vi "RT Driver_Set Date And Time.vi"(4 "Password":string, 6 "User name":string, 8 "error in (no error)":errorcluster, 9 "Configuration":T1={"Server IP Address"="206.246.122.250", "UDP Port"=123, "Synchronization Interval"=60.0, "Synchronization Threshold"=0.01, "Debug Output Strings"=TRUE, "Maximum Offset To Apply"=0.0}, 10 "New time zone (Leave blank to keep current time zone)":string, 11 "Correction (S/s)":dbl) -> (0 "error out":errorcluster)   [LabVIEW 2013, in "SNTP Light Custom Device Engine.lvlib"]
uses:
  SNTP Light Custom Device Engine.lvlib
  RT_Configuration_Data.ctl
  RT Driver_Global.vi
  <vilib>/nisyscfg/nisyscfg.lvlib
  <vilib>/NI_Real-Time Target Support.lvlib
  <vilib>/NI Veristand/Custom Device Tools/Custom Device Utility Library/Custom Device Utility Library.lvlib
panel:
  out "New Time":timestamp format="%<%.6X\n%x>T"
  out "current time":timestamp format="%<%.6X\n%x>T"
  out "Last Correction (s)":dbl
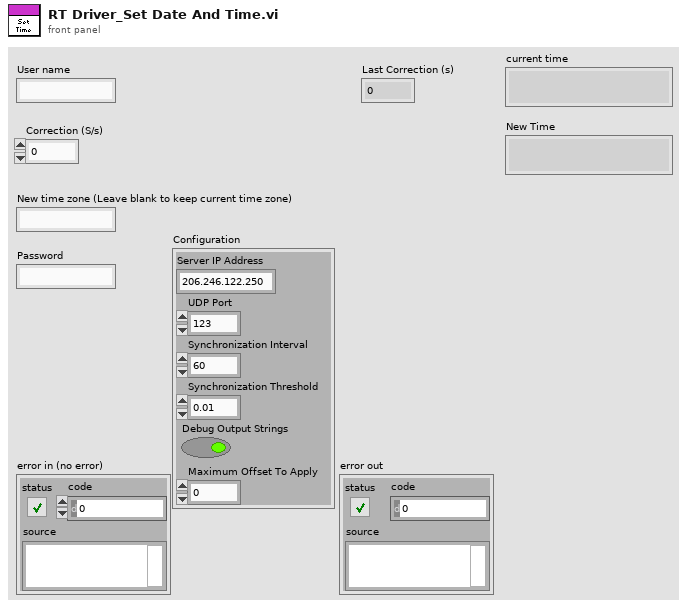
[diagram p1: front panel]
types:
  T1 = typedef "SNTP Light Custom Device Engine.lvlib/RT_Configuration_Data.ctl" = cluster{"Server IP Address":string, "UDP Port":u16, "Synchronization Interval":dbl, "Synchronization Threshold":dbl, "Debug Output Strings":bool, "Maximum Offset To Apply":dbl}
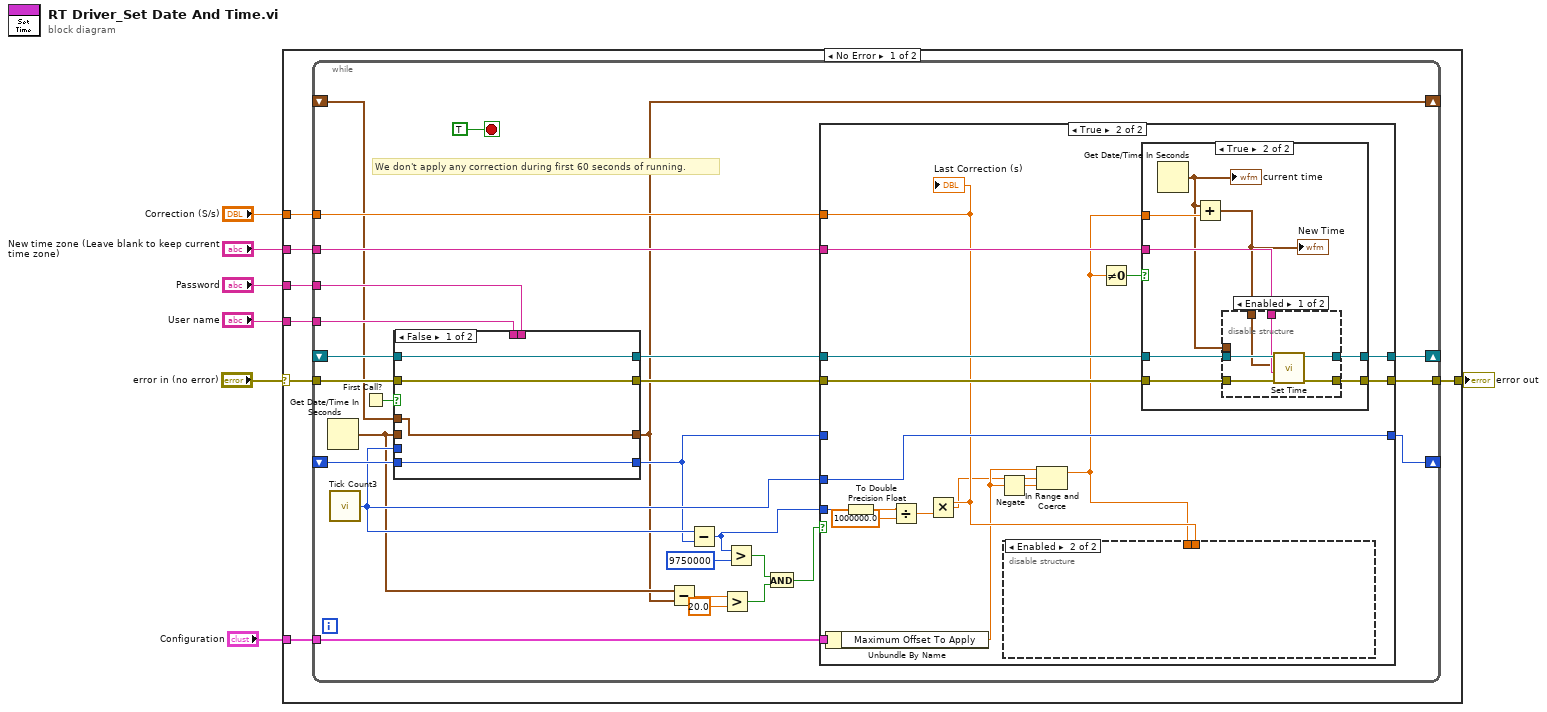
[diagram p0: block diagram]
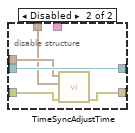
[diagram p4: hidden frame]
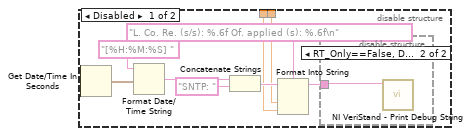
[diagram p5: hidden frame]
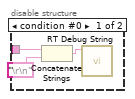
[diagram p6: hidden frame]
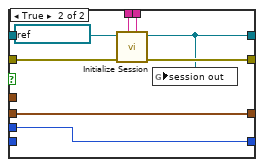
[diagram p7: hidden frame]
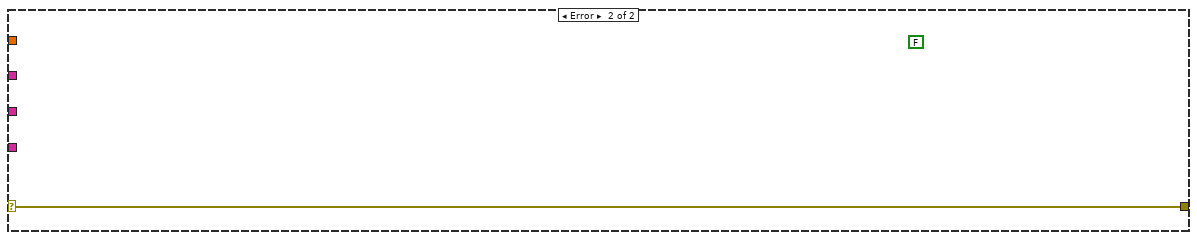
[diagram p8: hidden frame]
diagram:
  n1 = case shown="No Error" "error in (no error)" {
    selector: "error in (no error)" -> [w10 w108]
    tunnel: [w14 w108] -> w7
    tunnel: "Password" -> [w13 _]
    tunnel: "User name" -> [w12 _]
    tunnel: "New time zone (Leave blank to keep current time zone)" -> [w11 _]
    tunnel: "Correction (S/s)" -> [w9 _]
    tunnel: "Configuration" -> [w8 _]
    frame No Error {
      n2 = while {
        tunnel: w11 -> [w39]
        tunnel: w12 -> [w38]
        tunnel: w13 -> [w37]
        tunnel: w10 -> [w36]
        tunnel: [w34] -> w14
        shift-right: [w33] -> _
        shift-left: _ -> [w32]
        tunnel: w9 -> [w30]
        shift-right: [w26] -> _
        shift-left: _ -> [w29]
        shift-right: [w21] -> _
        shift-left: _ -> [w23]
        tunnel: w8 -> [w15]
        stop <- TRUE stop-if-true
        # "We don't apply any correction during first 60 seconds of running."
        n3 = Get Date/Time In Seconds() -> (seconds since 1Jan1904=w22:timestamp)
        n4 = call "Tick Count3"() -> ("Tick Count(uSec)"=w28:u32)
        n5 = First Call?() -> (First Call?: T/F=w31:bool)
        n6 = case shown="False" w31 {
          tunnel: [w99 w102] -> w41
          tunnel: [w98 w107] -> w40
          tunnel: w38 -> [_ w106]
          tunnel: w37 -> [_ w105]
          tunnel: w36 -> [w98 w103]
          tunnel: w32 -> [w99 _]
          tunnel: w29 -> [w97 _]
          tunnel: [w97 w101] -> w27
          tunnel: w28 -> [_ w101]
          tunnel: [w96 w100] -> w21
          tunnel: w22 -> [_ w100]
          tunnel: w23 -> [w96 _]
          frame False {
          }
          frame True {
            n7 = call <vilib>:"Initialize Session.vi"("password"=w105, "user name"=w106, "error in (no error)"=w103, "target (localhost)"=refnum<k21> "localhost" ("Target")) -> ("error out"=w107:errorcluster, "session out"=w102:refnum<k21>)  [unwired: 6 in]
            n8 = global write "RT Driver_Global.vi" "session out"(w102) -> ()
          }
        }
        n9 = Subtract(x=w22, y=w21) -> (x-y=w17:dbl)
        n10 = Subtract(x=w28, y=w27) -> (x-y=w24:u32)
        n11 = Greater?(x=w17, y=20.0) -> (0:w18:bool)
        n12 = Greater?(x=w24, y=u32 9750000) -> (0:w20:bool)
        n13 = And(x=w20, y=w18) -> (x .and. y?=w19:bool)
        n14 = case shown="True" w19 {
          tunnel: w41 -> [w43 w61]
          tunnel: w40 -> [w42 w60]
          tunnel: w39 -> [_ w59]
          tunnel: [w42 w58] -> w34
          tunnel: [w43 w57] -> w33
          tunnel: w28 -> [_ w56]
          tunnel: w27 -> [w44 _]
          tunnel: [w44 w56] -> w26
          tunnel: w24 -> [_ w55]
          tunnel: w30 -> [_ w52]
          tunnel: w15 -> [_ w50]
          frame False {
          }
          frame True {
            n15 = Unbundle By Name(w50) -> ("Maximum Offset To Apply"=w48:dbl)
            n16 = To Double Precision Float(number=w55) -> (double precision float=w53:dbl)
            n17 = Divide(x=w53, y=1000000.0) -> (x/y=w51:dbl)
            n18 = Multiply(x=w52, y=w51) -> (x*y=w46:dbl)
            n19 = Negate(x=w48) -> (-x=w49:dbl)
            n20 = In Range and Coerce(upper limit=w48, x=w46, lower limit=w49) -> (coerced(x)=w45:dbl)  [unwired: 1 out]
            n21 = disable-structure shown="Enabled" {
              disable-tunnel: w52 -> [w85 _]
              disable-tunnel: w45 -> [w84 _]
              frame Disabled {
                n22 = Get Date/Time In Seconds() -> (seconds since 1Jan1904=w87:timestamp)
                n23 = Format Date/Time String(time format string (%c)="[%H:%M:%S] ", seconds (now)=w87) -> (date/time string=w90:string)  [unwired: 1 in]
                n24 = Concatenate Strings(w90, "SNTP: " ("initial string")) -> (w91:string)
                n25 = Format Into String(format string="L. Co. Re. (s/s): %.6f Of. applied (s): %.6f\n", initial string=w91, w85, w84) -> (resulting string=w86:string)  [unwired: 1 in, 1 out]
                n26 = disable-structure shown="RT_Only==False, Default" {
                  disable-tunnel: w86 -> [w94 w95]
                  frame condition #0 {
                    n27 = Concatenate Strings(w94, "\r\n") -> (w93:string)
                    n28 = call <vilib>:"RT Debug String.vi"("String to write"=w93) -> ()  [unwired: 10 in, 1 out]
                  }
                  frame condition #1 (active) {
                    n29 = call <vilib>:"NI VeriStand - Print Debug String.vi"("Message"=w95) -> ()  [unwired: 10 in, 1 out]
                  }
                }
              }
              frame Enabled {
              }
            }
            n30 = Not Equal To 0?(x=w45) -> (x != 0?=w47:bool)
            n31 = case shown="True" w47 {
              tunnel: w61 -> [w63 w71]
              tunnel: w60 -> [w62 w70]
              tunnel: w59 -> [_ w69]
              tunnel: [w62 w67] -> w58
              tunnel: [w63 w66] -> w57
              tunnel: w45 -> [_ w65]
              frame False {
              }
              frame True {
                n32 = Get Date/Time In Seconds() -> (seconds since 1Jan1904=w64:timestamp)
                "current time" <- w64
                n33 = Add(x=w64, y=w65) -> (x+y=w68:timestamp)
                "New Time" <- w68
                n34 = disable-structure shown="Enabled" {
                  disable-tunnel: w71 -> [w77 w82]
                  disable-tunnel: w70 -> [w76 w81]
                  disable-tunnel: w69 -> [w75 _]
                  disable-tunnel: w68 -> [w74 w78]
                  disable-tunnel: [w73 w80] -> w67
                  disable-tunnel: [w72 w82] -> w66
                  disable-tunnel: w64 -> [_ w79]
                  frame Enabled {
                    n35 = call <vilib>:"Set Time.vi"("error in (no error)"=w76, "time zone"=w75, "time"=w74, "session in (localhost)"=w77) -> ("error out"=w73:errorcluster, "session out"=w72:refnum<k21>)  [unwired: 4 in, 2 out]
                  }
                  frame Disabled {
                    n36 = call <vilib>:"TimeSyncAdjustTime.vi"("error in"=w81, "masterTime"=w78, "slaveTime"=w79) -> ("error out"=w80:errorcluster)  [unwired: 8 in]
                  }
                }
              }
            }
            "Last Correction (s)" <- w52
          }
        }
      }
    }
    frame Error {
      (unwired) FALSE ("changes require restart")
    }
  }
  "error out" <- w7
